vi "MeasureDriveAcceleration.vi"(2 "Average Drive Velocity (ft/s)":dbl(slide) scale=0.0..15.0, 4 "Reset":bool) -> (5 "Acceleration (ft/s^2)":dbl format="%.1f")   [LabVIEW 2020]
doc: "This VI allows a the maximum robot acceleration (from a dead-stop) to be measured."
uses:
  1271c85c-7527-42a4-87cd-beef602def8c.vi
  4f773a67-0122-4639-853c-a990835ad9f9.vi
  f4d4cb4f-03fc-4c90-a25c-6a27675242c6.vi
  fb03bb82-eb29-4926-bd44-4320e3a910e4.vi
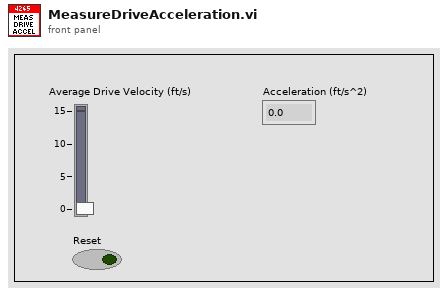
[diagram p1: front panel]
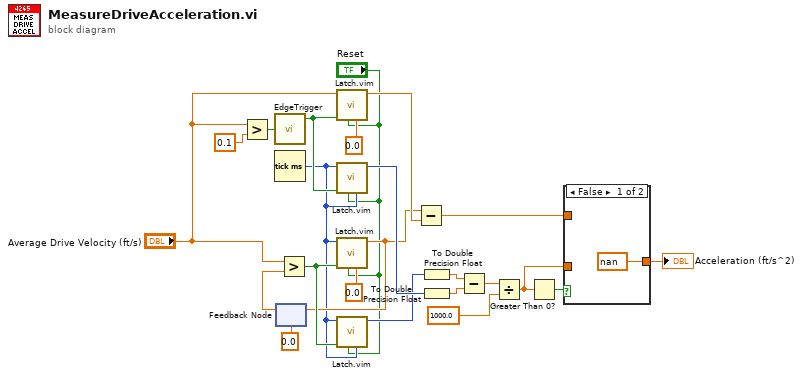
[diagram p0: block diagram]
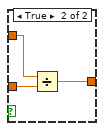
[diagram p2: hidden frame]
diagram:
  n1 = Greater?(x="Average Drive Velocity (ft/s)", y=0.1) -> (0:w8:bool)
  n2 = call "EdgeTrigger.vi"("Input Signal"=w8) -> ("Rising Edge Trigger"=w11:bool)  [unwired: 2 out]
  n3 = Tick Count (ms)() -> (millisecond timer value=w2:u32)
  n4 = feedback #1(0.0) -> (w4:dbl)
  n5 = Greater?(x="Average Drive Velocity (ft/s)", y=w4) -> (0:w6:bool)
  n6 = call "Latch.vim"("Default Value"=0.0, "Reset"="Reset", "Latch Signal"=w11, "Latch Value"="Average Drive Velocity (ft/s)") -> ("Latched"=w13:dbl)  [unwired: 7 in]
  n7 = call "Latch.vim"("Default Value"=w2, "Reset"="Reset", "Latch Signal"=w11, "Latch Value"=w2) -> ("Latched"=w15:u32)  [unwired: 7 in]
  n8 = call "Latch.vim"("Default Value"=0.0, "Reset"="Reset", "Latch Signal"=w6, "Latch Value"=w2) -> ("Latched"=w3:dbl)  [unwired: 7 in]
  n9 = feedback-in #1(w3) -> ()
  n10 = call "Latch.vim"("Default Value"=w2, "Reset"="Reset", "Latch Signal"=w6, "Latch Value"=w2) -> ("Latched"=w14:u32)  [unwired: 7 in]
  n11 = Subtract(x=w3, y=w13) -> (x-y=w22:dbl)
  n12 = To Double Precision Float(number=w14) -> (double precision float=w16:dbl)
  n13 = To Double Precision Float(number=w15) -> (double precision float=w17:dbl)
  n14 = Subtract(x=w16, y=w17) -> (x-y=w18:dbl)
  n15 = Divide(x=w18, y=1000.0) -> (x/y=w21:dbl)
  n16 = Greater Than 0?(x=w21) -> (x > 0?=w20:bool)
  n17 = case shown="False" w20 {
    tunnel: w21 -> [_ w27]
    tunnel: w22 -> [_ w26]
    tunnel: [nan w25] -> w23
    frame False {
    }
    frame True {
      n18 = Divide(x=w26, y=w27) -> (x/y=w25:dbl)
    }
  }
  "Acceleration (ft/s^2)" <- w23
